vi "PCO_GetLensFocus.vi"(8 "error in (no error)":errorcluster {"code" format="%x"}, 11 "hLens":u64) -> (0 "error out":errorcluster {"code" format="%x"}, 1 "lFocusPos":i32, 2 "ErrorMessage":i32 format="%x", 3 "hLens out":u64, 5 "dwflags":u32)   [LabVIEW 2019, in "SDK.lvlib" / "LensControl.lvlib"]
doc: "<b>Description:</b>\nGets the current focus of the lens control device as value between 0...0x3FFF.\n\n<b>Supported camera type:</b>\npco.edge CLHS, pco.dimax cs\n\n<b>Descriptor dependency:</b>\nNone"
uses:
  LensControl.lvlib
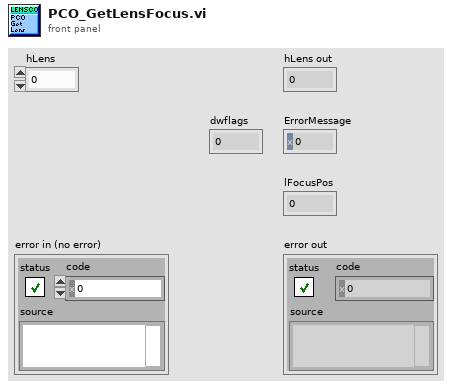
[diagram p1: front panel]
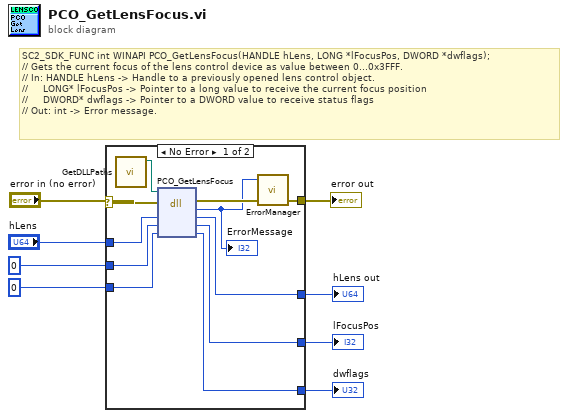
[diagram p0: block diagram]
diagram:
  # "SC2_SDK_FUNC int WINAPI PCO_GetLensFocus(HANDLE hLens, LONG *lFocusPos, DWORD *dwflags);\n// Gets the current focus of the lens control device as value between 0...0x3FFF.\n// In: HANDLE hLens -> Handle to a previously opened lens control object.\n//     LONG* lFocusPos -> Pointer to a long value to receive the current focus position\n//     DWORD* dwflags -> Pointer to a DWORD value to receive status flags\n// Out: int -> Error message."
  n1 = case shown="No Error" "error in (no error)" {
    selector: "error in (no error)" -> [w13 w23]
    tunnel: "hLens" -> [w19 w22]
    tunnel: [w18 w22] -> w7
    tunnel: 0 ("lFocusPos") -> [w17 w21]
    tunnel: [w16 w21] -> w5
    tunnel: u32 0 ("dwflags") -> [w15 w20]
    tunnel: [w14 w20] -> w3
    tunnel: [w12 w23] -> w2
    frame No Error {
      n2 = call "GetDLLPaths.vi"() -> ("SC2_Cam_Path"=w9:path)  [unwired: 8 in, 3 out]
      n3 = dll-call lib="?" fn="PCO_GetLensFocus"(path in=w9, error in=w13, "hLens"=w19, "lFocusPos"=w17, "dwflags"=w15) -> (error out=w11:errorcluster, "return type"=w10:i32, "hLens"=w18:u64, "lFocusPos"=w16:i32, "dwflags"=w14:u32)  [unwired: 1 in, 1 out]
      "ErrorMessage" <- w10
      n4 = call "ErrorManager.vi"("error in (no error)"=w11, "error code"=w10) -> ("error out"=w12:errorcluster)  [unwired: 2 in, 1 out]
    }
    frame Error {
    }
  }
  "hLens out" <- w7
  "lFocusPos" <- w5
  "dwflags" <- w3
  "error out" <- w2
